vi "Replace Constant with XNode.vi"(4 "Error In":errorcluster, 6 "Const Ref":refnum<vi>, 7 "XRef":T1) -> (0 "Error Out":errorcluster)   [LabVIEW 2025, in "XNode Support.lvlib"]
doc: "Connects the XNode to the Constant's connected wire, then deletes the Constant"
uses:
  XNode Support.lvlib
  <vilib>/XNodeSupport/XNodeXNodeRef.ctl
  <vilib>/XNodeSupport/NI_XNodeSupport.lvlib
panel:
  out "dup XRef":T1
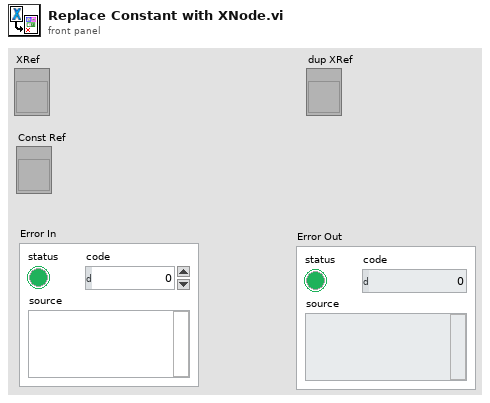
[diagram p1: front panel]
types:
  T1 = typedef "NI_XNodeSupport.lvlib/XNodeXNodeRef.ctl" = refnum<vi>
  T2 = typedef "LVRectTypeDef.ctl" = cluster{"Left":i16, "Top":i16, "Right":i16, "Bottom":i16}
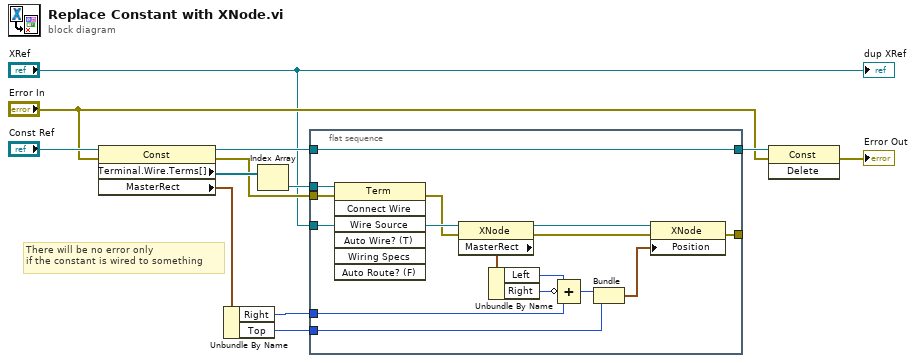
[diagram p0: block diagram]
diagram:
  # "There will be no error only\nif the constant is wired to something"
  n1 = property class="Const"(reference="Const Ref", error in="Error In") -> (reference out=w10:refnum<vi>, error out=w8:errorcluster, "Terminal.Wire.Terms[]"=w11:refnum<vi>[], "MasterRect"=w3:T2)
  n2 = Unbundle By Name(w3) -> ("Right"=w2:i16, "Top"=w1:i16)
  n3 = Index Array(array=w11) -> (element=w12:refnum<vi>)  [unwired: 1 in]
  n4 = flat-sequence {
    tunnel: "XRef" -> [w17]
    tunnel: w12 -> [w27]
    tunnel: w8 -> [w26]
    tunnel: w10 -> [w25]
    tunnel: [w25] -> w9
    tunnel: [w24] -> _
    tunnel: w2 -> [w14]
    tunnel: w1 -> [w20]
    frame #0 {
      n5 = invoke class="Term" method="Connect Wire"(reference=w27, error in=w26, "Wire Source"=w17) -> (error out=w16:errorcluster)  [unwired: 4 in, 6 out]
      n6 = property class="XNode"(reference=w17, error in=w16) -> (reference out=w18:T1, error out=w15:errorcluster, "MasterRect"=w23:T2)
      n7 = Unbundle By Name(w23) -> ("Left"=w13:i16, "Right"=w22:i16)
      n8 = Compound Arithmetic op=ADD(w13, invert w22, w14) -> (w21:i16)
      n9 = Bundle(w21, "Top"=w20) -> (w19:cluster{i16, "Top":i16})  [unwired: 1 in]
      n10 = property class="XNode"(reference=w18, error in=w15, "Position"=w19) -> (error out=w24:errorcluster)  [unwired: 1 out]
    }
  }
  n11 = invoke class="Const" method="Delete"(reference=w9, error in="Error In") -> (error out=→"Error Out":errorcluster)  [unwired: 1 in, 2 out]
  "dup XRef" <- "XRef"
